vi "TopasExample.vi"() -> ()   [LabVIEW 2017]
panel:
  out "CallerHasAccess":bool
  in  "Shutter":bool
  in  "Interaction":string
  out "Progress":dbl(slide)=1.0 scale=0.0..1.0
  out "Wavelength Status":bool
  in  "Get Wavelength Button":bool
  in  "Wavelength, nm":dbl
  in  "Set Wavelength Button":bool
  out "Status":bool
  out "Available interactions":cluster{"Type":string, "From":dbl, "To":dbl}[](array[cluster])
  in  "Interactions Button":bool
  in  "Serial NUmber":string="Orpheus-HP-Demo-8047"
  in  "Cancel Button":bool
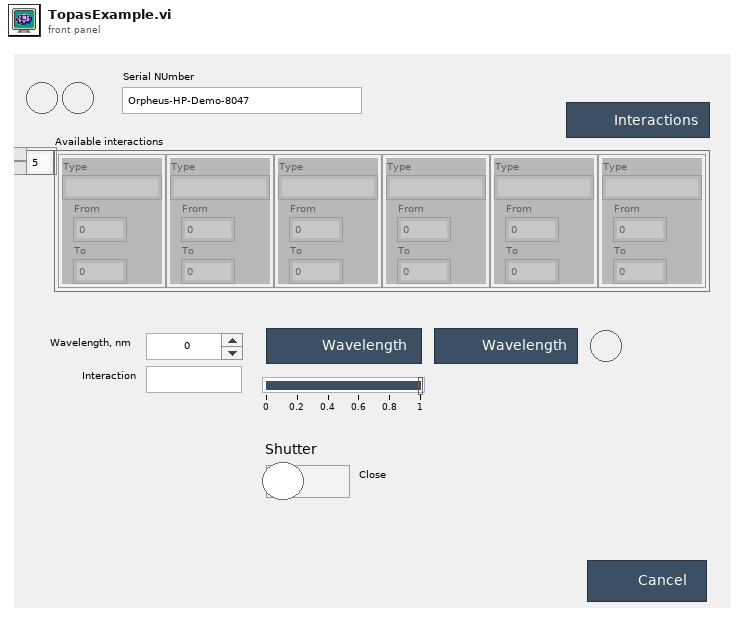
[diagram p1: front panel]
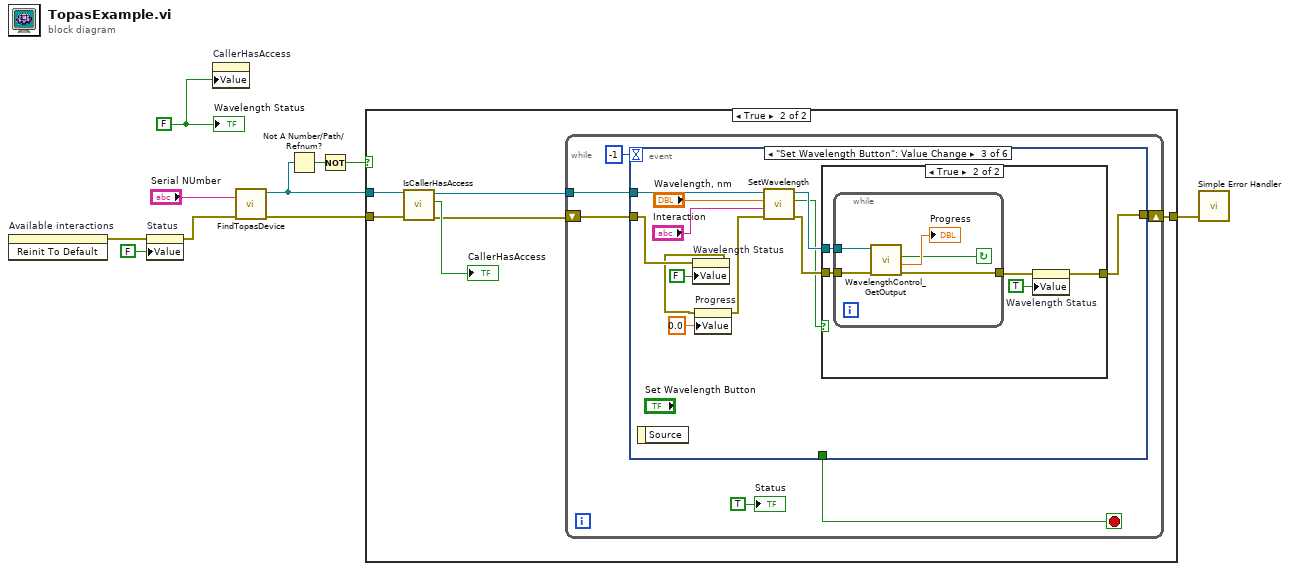
[diagram p0: block diagram]
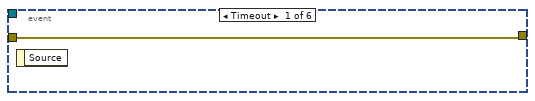
[diagram p3: hidden frame]
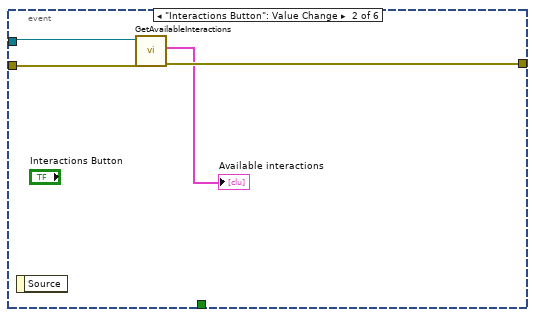
[diagram p4: hidden frame]
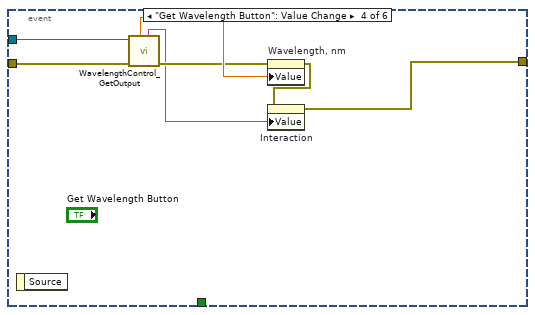
[diagram p6: hidden frame]
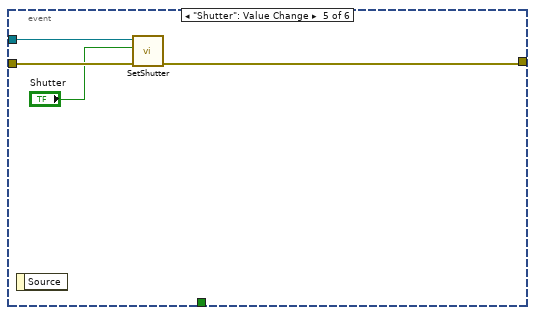
[diagram p7: hidden frame]
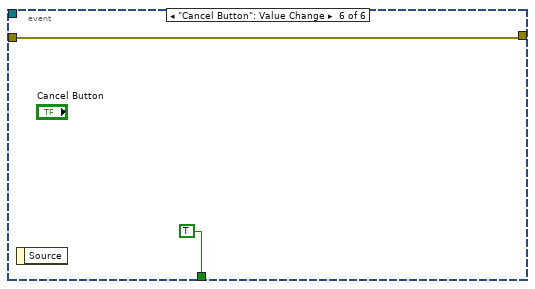
[diagram p8: hidden frame]
diagram:
  w1 = FALSE ("Wavelength Status")
  n1 = invoke on="Available interactions" class="Arr (strict)" method="Reinit To Default"() -> (error out=w5:errorcluster)  [unwired: 3 in, 2 out]
  n2 = property on="Status" class="Bool (strict)"(error in=w5, "Value"=FALSE ("Visible")) -> (error out=w6:errorcluster)  [unwired: 1 in, 1 out]
  n3 = property on="CallerHasAccess" class="Bool (strict)"("Value"=w1) -> ()  [unwired: 2 in, 2 out]
  n4 = call "FindTopasDevice.vi"("error in (no error)"=w6, "Serial number"="Serial NUmber") -> ("error out"=w9:errorcluster, "TopasDevice"=w4:refnum<k24>)  [unwired: 8 in]
  n5 = Not A Number/Path/Refnum?(number/path/refnum=w4) -> (NaN/Path/Refnum?=w3:bool)
  n6 = Not(x=w3) -> (.not. x?=w2:bool)
  n7 = case shown="True" w2 {
    tunnel: w9 -> [w11 w15]
    tunnel: [w11 w17] -> w8
    tunnel: w4 -> [_ w16]
    frame False {
    }
    frame True {
      n8 = call "IsCallerHasAccess.vi"("error in (no error)"=w15, "Topas"=w16) -> ("error out"=w12:errorcluster, "GetCallerHasAccess"=→"CallerHasAccess":bool, "Topas out"=w14:refnum<k24>)  [unwired: 7 in]
      n9 = while {
        tunnel: w14 -> [w22]
        shift-right: [w20] -> w17
        shift-left: w12 -> [w21]
        stop <- w19 stop-if-true
        n10 = event shown="[2] \"Set Wavelength Button\": Value Change" {
          selector: _ -> [_ _ _ _ _ _]
          dyn-events: _ -> [_ _ _ _ _ _]
          timeout: -1 -> [_ _ _ _ _ _]
          tunnel: w22 -> [_ w26 w40 w58 w62 _]
          tunnel: w21 -> [w24 w28 w38 w57 w61 w64]
          tunnel: [w24 w27 w36 w52 w60 w64] -> w20
          tunnel: [_ _ _ _ _ TRUE] -> w19
          event Timeout {
            n11 = event-data() -> ()  [unwired: 1 in, 1 out]
          }
          event "Interactions Button": Value Change {
            n12 = event-data() -> ()  [unwired: 1 in, 1 out]
            n13 = call "GetAvailableInteractions.vi"("error in (no error)"=w28, "Topas In"=w26) -> ("error out"=w27:errorcluster, "Available interactions"=→"Available interactions":cluster{"Type":string, "From":dbl, "To":dbl}[])  [unwired: 7 in, 1 out]
          }
          event "Set Wavelength Button": Value Change {
            n14 = event-data() -> ()  [unwired: 1 in, 1 out]
            n15 = property on="Wavelength Status" class="Bool (strict)"(error in=w38, "Value"=FALSE ("Wavelength Status")) -> (error out=w34:errorcluster)  [unwired: 1 in, 1 out]
            n16 = property on="Progress" class="Slide (strict)"(error in=w34, "Value"=0.0 ("Progress")) -> (error out=w33:errorcluster)  [unwired: 1 in, 1 out]
            n17 = call "SetWavelength.vi"("error in (no error)"=w33, "Interaction Type"="Interaction", "Wavelength, nm"="Wavelength, nm", "Topas In"=w40) -> ("error out"=w31:errorcluster, "IsSuccess"=w29:bool, "Topas out"=w32:refnum<k24>)  [unwired: 5 in]
            n18 = case shown="True" w29 {
              tunnel: [w41 w46] -> w36
              tunnel: w32 -> [_ w45]
              tunnel: w31 -> [w41 w44]
              frame False {
              }
              frame True {
                n19 = while {
                  tunnel: w45 -> [w50]
                  tunnel: w44 -> [w48]
                  tunnel: [w47] -> w43
                  stop <- w49 continue-if-true
                  n20 = call "WavelengthControl_GetOutput.vi"("error in (no error)"=w48, "Topas"=w50) -> ("error out"=w47:errorcluster, "WavelengthSettingCompletionPart"=→"Progress":dbl, "IsWavelengthSettingInProgress"=w49:bool)  [unwired: 4 in, 3 out]
                }
                n21 = property on="Wavelength Status" class="Bool (strict)"(error in=w43, "Value"=TRUE ("Wavelength Status")) -> (error out=w46:errorcluster)  [unwired: 1 in, 1 out]
              }
            }
          }
          event "Get Wavelength Button": Value Change {
            n22 = event-data() -> ()  [unwired: 1 in, 1 out]
            n23 = call "WavelengthControl_GetOutput.vi"("error in (no error)"=w57, "Topas"=w58) -> ("error out"=w55:errorcluster, "Interaction"=w54:string, "Wavelength"=w56:dbl)  [unwired: 4 in, 3 out]
            n24 = property on="Wavelength, nm" class="DigNum (strict)"(error in=w55, "Value"=w56) -> (error out=w53:errorcluster)  [unwired: 1 in, 1 out]
            n25 = property on="Interaction" class="Str"(error in=w53, "Value"=w54) -> (error out=w52:errorcluster)  [unwired: 1 in, 1 out]
          }
          event "Shutter": Value Change {
            n26 = event-data() -> ()  [unwired: 1 in, 1 out]
            n27 = call "SetShutter.vi"("error in (no error)"=w61, "State"="Shutter", "Topas"=w62) -> ("error out"=w60:errorcluster)  [unwired: 7 in, 1 out]
          }
          event "Cancel Button": Value Change {
            n28 = event-data() -> ()  [unwired: 1 in, 1 out]
          }
        }
        "Status" <- TRUE ("Status")
      }
    }
  }
  n29 = call <vilib>:"Simple Error Handler.vi"("error in (no error)"=w8) -> ()  [unwired: 4 in, 5 out]
  "Wavelength Status" <- w1
